vi "tsdiag_can_security_access_send_key.vi"(6 "AKeyValue":u8[](array[numeric]), 8 "错误输入（无错误）":errorcluster, 9 "ALevel":i32, 10 "ADiagModuleIndex":i32, 11 "path":path) -> (0 "错误输出":errorcluster, 2 "Return Type":i32, 3 "path out":path)   [LabVIEW 2014]
doc: "Function Introduction :\n27 key send key\nCall location :\nAfter connecting the hardware, it is no longer necessary to create a diagnostic module\ninput parameter :\nADiagModulus Index: Handle to UDS module\nALevel: Security Level\nAKeyValue: A data pointer used to store key values AKeySize: Key value size\nReturn value :\n==0: Execution successful\nOther values: Query error code"
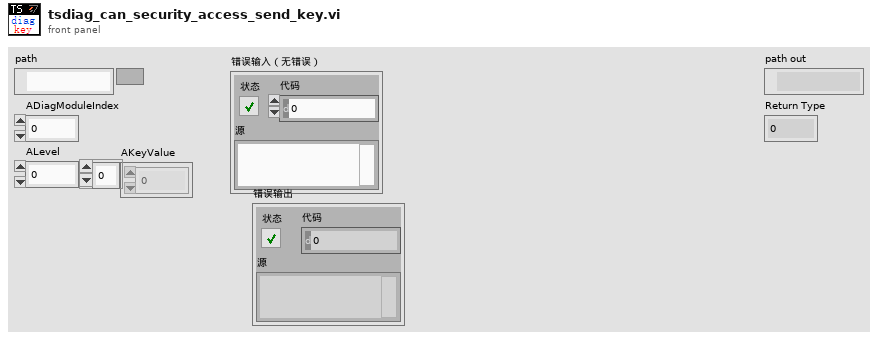
[diagram p1: front panel]
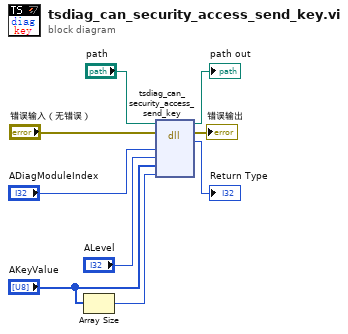
[diagram p0: block diagram]
diagram:
  n1 = Array Size(array="AKeyValue") -> (size(s)=w4:i32)
  n2 = dll-call lib="C:/Users/XYY/Desktop/LabView Demo/TSCAN_LB2018_V1.4_20220309/Config/TSMaster.dll" fn="tsdiag_can_security_access_send_key"(path in="path", error in="错误输入（无错误）", "ADiagModuleIndex"="ADiagModuleIndex", "ALevel"="ALevel", "AKeyValue"="AKeyValue", "AKeySize"=w4) -> (path out=→"path out":path, error out=→"错误输出":errorcluster, "返回类型"=→"Return Type":i32)  [unwired: 5 in]
